vi "debug_webdav_1.vi"() -> ()   [LabVIEW 2014]
uses:
  <vilib>/WebDAVClient/Advanced/FileInfo.ctl
  <vilib>/WebDAVClient/NI_WebDAV.lvlib
panel:
  out "date string":string
  out "directory list":T1[](array[typedef])
  out "error out":errorcluster
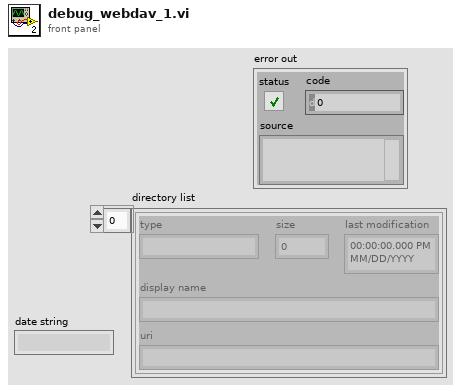
[diagram p1: front panel]
types:
  T1 = typedef "NI_WebDAV.lvlib/FileInfo.ctl" = cluster{"type":string, "size":u64, "last modification":timestamp, "display name":string, "uri":string}
  T2 = typedef "NI_WebDAV.lvlib/SessionHandle.ctl" = refnum<k1>
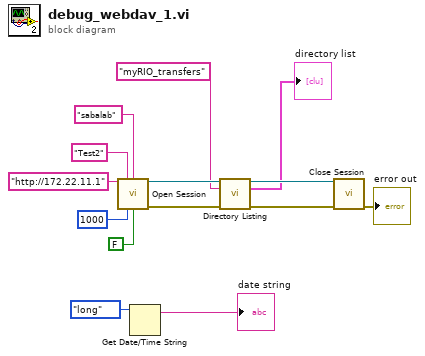
[diagram p0: block diagram]
diagram:
  n1 = call <vilib>:"Open Session.vi"("host uri prefix"="http://172.22.11.1", "username"="Test2", "password"="sabalab", "timeout ms"=1000, "verify server?"=FALSE) -> ("session handle out"=w9:T2, "error out"=w7:errorcluster)  [unwired: 9 in]
  n2 = Get Date/Time String(date format (0)=enum16{"short", "long", "abbreviated"}."long") -> (date string=→"date string":string)  [unwired: 2 in, 1 out]
  n3 = call <vilib>:"Directory Listing.vi"("session handle"=w9, "relative uri"="myRIO_transfers", "error in (no error)"=w7) -> ("session handle out"=w8:T2, "directory list"=→"directory list":T1[], "error out"=w6:errorcluster)  [unwired: 9 in, 1 out]
  n4 = call <vilib>:"Close Session.vi"("session handle"=w8, "error in (no error)"=w6) -> ("error out"=→"error out":errorcluster)  [unwired: 13 in]
